vi "Is a Corner.vi"(3 "Corner candidate":cluster{"Col":dbl, "Row":dbl}, 4 "Updated Map":T1) -> (1 "Is a corner":bool)   [LabVIEW 2009]
uses:
  <vilib>/Analysis/Matrix/Datatypes/RealMatrix.ctl
  <vilib>/Analysis/Matrix/NI_Matrix.lvlib
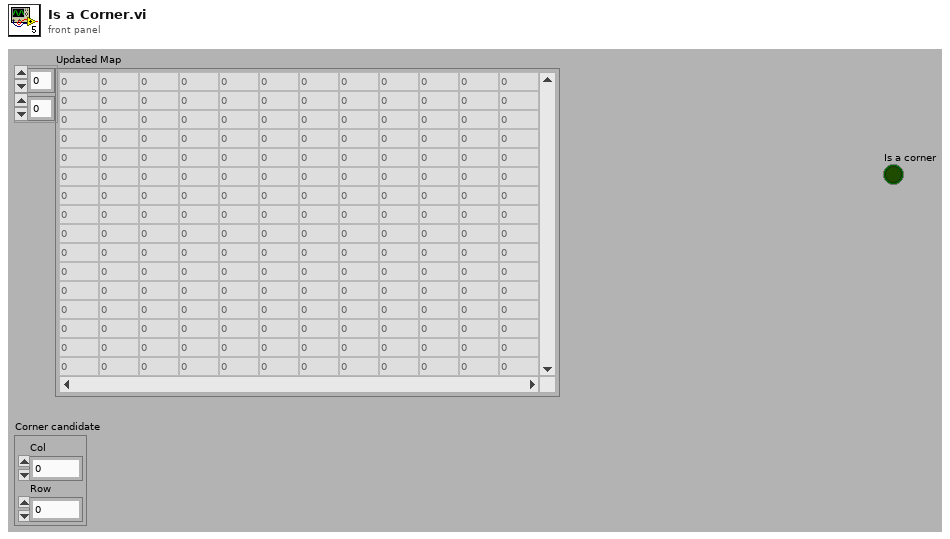
[diagram p1: front panel]
types:
  T1 = typedef "NI_Matrix.lvlib/RealMatrix.ctl" = dbl[][]
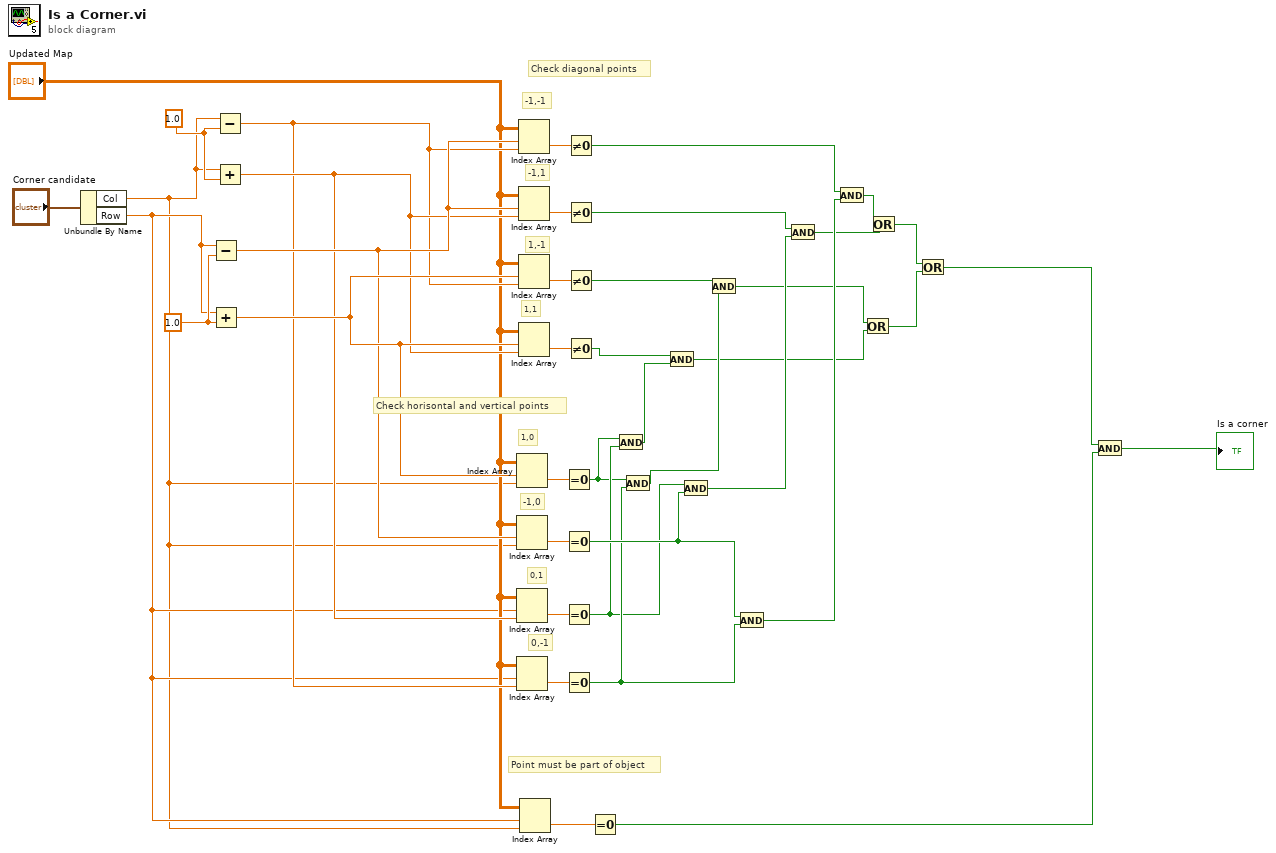
[diagram p0: block diagram]
diagram:
  w34 = 1.0 ("x")
  w40 = 1.0 ("y")
  # "1,1"
  # "1,-1"
  # "-1,1"
  # "-1,-1"
  # "0,-1"
  # "0,1"
  # "-1,0"
  # "1,0"
  # "Point must be part of object"
  # "Check horisontal and vertical points"
  # "Check diagonal points"
  n1 = Unbundle By Name("Corner candidate") -> ("Col"=w23:dbl, "Row"=w24:dbl)
  n2 = Subtract(x=w24, y=w40) -> (x-y=w28:dbl)
  n3 = Add(x=w24, y=w40) -> (x+y=w29:dbl)
  n4 = Subtract(x=w23, y=w34) -> (x-y=w26:dbl)
  n5 = Add(x=w23, y=w34) -> (x+y=w27:dbl)
  n6 = Index Array(array="Updated Map", index (row)=w29, index (col)=w23) -> (element=w33:dbl)
  n7 = Index Array(array="Updated Map", index (row)=w28, index (col)=w23) -> (element=w32:dbl)
  n8 = Index Array(array="Updated Map", index (row)=w24, index (col)=w27) -> (element=w31:dbl)
  n9 = Index Array(array="Updated Map", index (row)=w24, index (col)=w26) -> (element=w30:dbl)
  n10 = Index Array(array="Updated Map", index (row)=w28, index (col)=w26) -> (element=w38:dbl)
  n11 = Index Array(array="Updated Map", index (row)=w28, index (col)=w27) -> (element=w37:dbl)
  n12 = Index Array(array="Updated Map", index (row)=w29, index (col)=w26) -> (element=w36:dbl)
  n13 = Index Array(array="Updated Map", index (row)=w29, index (col)=w27) -> (element=w35:dbl)
  n14 = Index Array(array="Updated Map", index (row)=w24, index (col)=w23) -> (element=w22:dbl)
  n15 = Equal To 0?(x=w33) -> (x = 0?=w11:bool)
  n16 = Equal To 0?(x=w32) -> (x = 0?=w18:bool)
  n17 = Equal To 0?(x=w31) -> (x = 0?=w12:bool)
  n18 = Equal To 0?(x=w30) -> (x = 0?=w15:bool)
  n19 = Not Equal To 0?(x=w38) -> (x != 0?=w21:bool)
  n20 = Not Equal To 0?(x=w37) -> (x != 0?=w19:bool)
  n21 = Not Equal To 0?(x=w36) -> (x != 0?=w16:bool)
  n22 = Not Equal To 0?(x=w35) -> (x != 0?=w13:bool)
  n23 = Equal To 0?(x=w22) -> (x = 0?=w2:bool)
  n24 = And(x=w11, y=w12) -> (x .and. y?=w10:bool)
  n25 = And(x=w11, y=w15) -> (x .and. y?=w14:bool)
  n26 = And(x=w13, y=w10) -> (x .and. y?=w6:bool)
  n27 = And(x=w12, y=w18) -> (x .and. y?=w17:bool)
  n28 = And(x=w16, y=w14) -> (x .and. y?=w7:bool)
  n29 = And(x=w18, y=w15) -> (x .and. y?=w20:bool)
  n30 = And(x=w19, y=w17) -> (x .and. y?=w8:bool)
  n31 = And(x=w21, y=w20) -> (x .and. y?=w9:bool)
  n32 = Or(x=w7, y=w6) -> (x .or. y?=w4:bool)
  n33 = Or(x=w9, y=w8) -> (x .or. y?=w5:bool)
  n34 = Or(x=w5, y=w4) -> (x .or. y?=w1:bool)
  n35 = And(x=w1, y=w2) -> (x .and. y?=→"Is a corner":bool)
